vi "Do.vi"(7 "Mediated Asynchronous Actor":refnum<class "Mediated Asynchronous Actor.lvclass">, 8 "error in (no error)":errorcluster, 11 "Remove Connected Client from WSserver Msg in":refnum<class "Remove Connected Client from WSserver Msg.lvclass">) -> (0 "error out":errorcluster, 3 "Remove Connected Client from WSserver Msg out":refnum<class "Remove Connected Client from WSserver Msg.lvclass">, 5 "Mediated Asynchronous Actor out":refnum<class "Mediated Asynchronous Actor.lvclass">)   [LabVIEW 2016, in "WebSocket Networking.lvlib" / "Remove Connected Client from WSserver Msg.lvclass"]
doc: "--\nCopyright © 2017 Composed SystemsI All rights reserved.\n\nAuthor: Jon McBee <jon.mcbee@composed.io>\n\nThis library is provided \"AS IS\" ,WITHOUT WARRANTIES OR\nCONDITIONS OF ANY KIND, either express or implied.\n\nComposed Systems -- composed.io\n\nStream 0.0.1.1\nJon McBee - Composed Systems\nCopyright (c) 2017, Composed Systems"
uses:
  <userlib>/Common Components/WebSocket Networking/WS Server Msgs/Remove Connected Client from WSserver Msg/Remove Connected Client from WSserver Msg.lvclass
  <userlib>/Composed Systems/Stream/Mediator/Classes/Mediated Asynchronous Actor/Mediated Asynchronous Actor.lvclass
  <userlib>/Common Components/WebSocket Networking/WS Server/WS Server.lvclass
  C:/Program Files (x86)/National Instruments/LabVIEW 2016/user.lib/Composed Systems/Stream/Mediator/Classes/Mediated Asynchronous Actor/Mediated Asynchronous Actor.lvclass
  <userlib>/Common Components/WebSocket Networking/WS Server Msgs/Remove Connected Client from WSserver Msg/Remove Connected Client from WSserver Msg.lvclass/Remove Connected Client from WSserver Msg.ctl
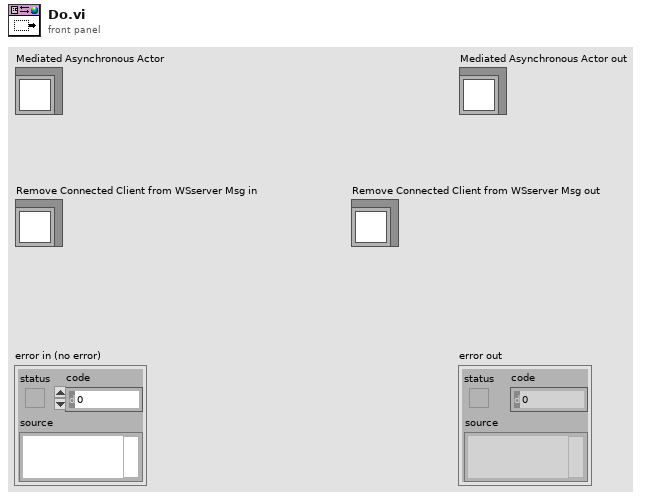
[diagram p1: front panel]
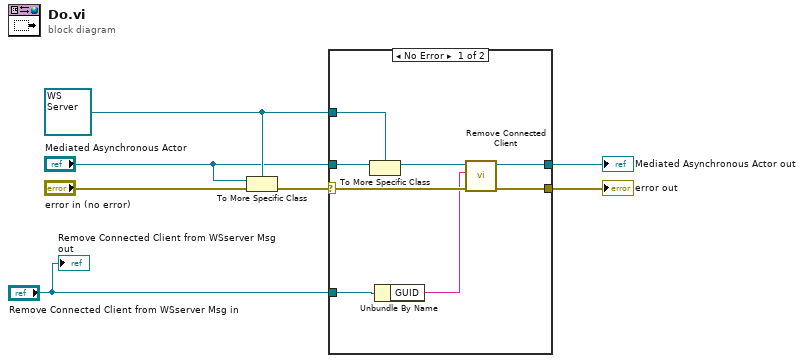
[diagram p0: block diagram]
diagram:
  w5 = refnum<class "WS Server.lvclass"> refnum ("Websocket Server.lvclass")
  n1 = To More Specific Class(target class=w5, reference="Mediated Asynchronous Actor", error in="error in (no error)") -> (error out=w7:errorcluster)  [unwired: 1 out]
  n2 = case shown="No Error" w7 {
    selector: w7 -> [w10 w16]
    tunnel: w5 -> [w15 _]
    tunnel: "Mediated Asynchronous Actor" -> [w14 w17]
    tunnel: "Remove Connected Client from WSserver Msg in" -> [w13 _]
    tunnel: [w11 w17] -> w3
    tunnel: [w9 w16] -> w2
    frame No Error {
      n3 = To More Specific Class(target class=w15, reference=w14) -> (specific class reference=w12:refnum<class "WS Server.lvclass">)  [unwired: 1 in, 1 out]
      n4 = Unbundle By Name(w13) -> ("GUID"=w8:string)
      n5 = call <userlib>:"Remove Connected Client.vi"("error in (no error)"=w10, "GUID"=w8, "Websocket Server in"=w12) -> ("error out"=w9:errorcluster, "Websocket Server out"=w11:refnum<class "WS Server.lvclass">)  [unwired: 7 in]
    }
    frame Error {
    }
  }
  "error out" <- w2
  "Mediated Asynchronous Actor out" <- w3
  "Remove Connected Client from WSserver Msg out" <- "Remove Connected Client from WSserver Msg in"
